vi "Ageing_Loop.vi"(6 "Step Array In":i32[](array[numeric]), 8 "Input Array 2":string[](array[string]), 9 "Input Array 1":string[](array[string])) -> (0 "Step Array Out":i32[](array[numeric]), 1 "True/False":i16, 2 "Output Array 2":string[](array[string]), 3 "Output Array 1":string[](array[string]))   [LabVIEW 2014]
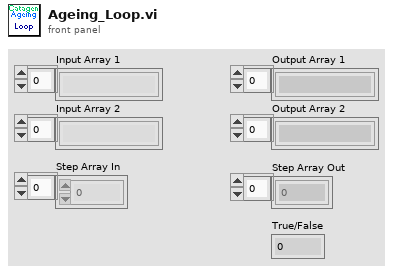
[diagram p1: front panel]
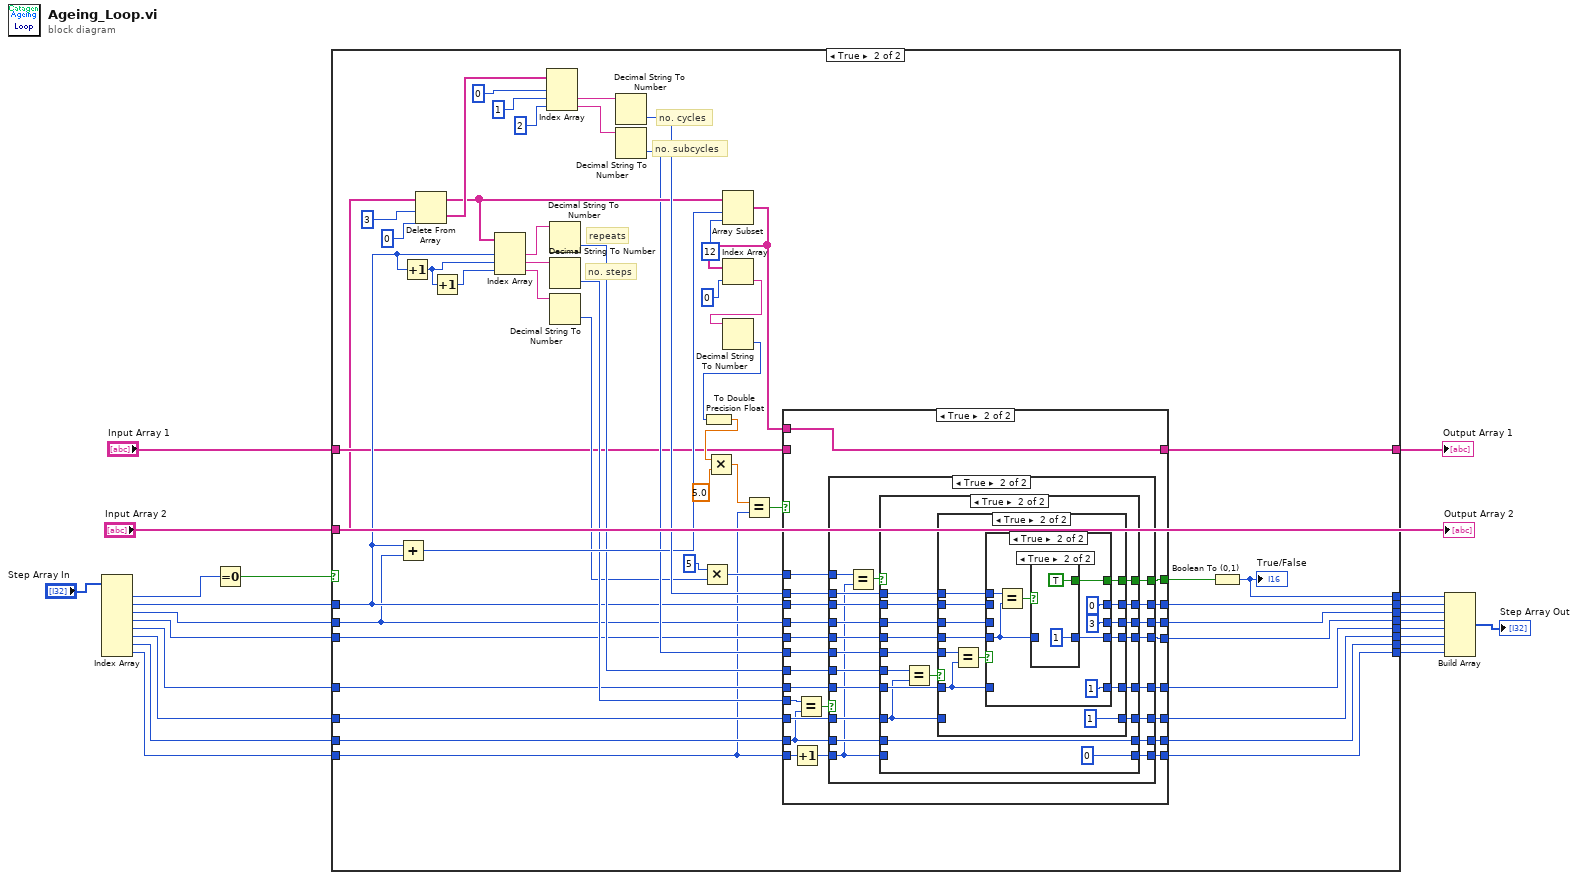
[diagram p0: block diagram]
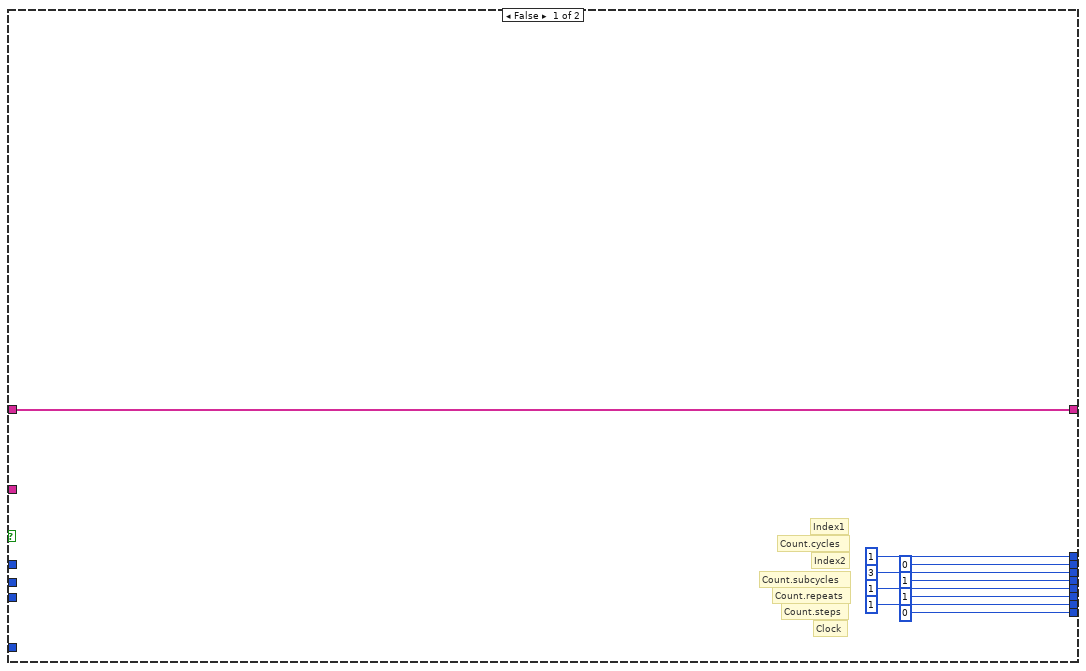
[diagram p2: hidden frame]
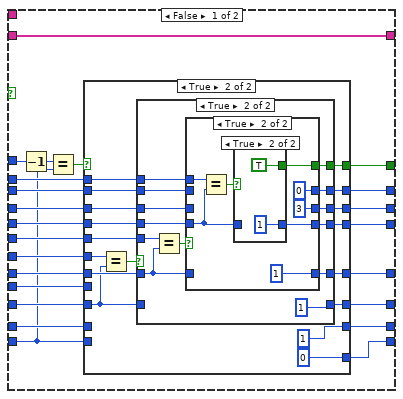
[diagram p3: hidden frame]
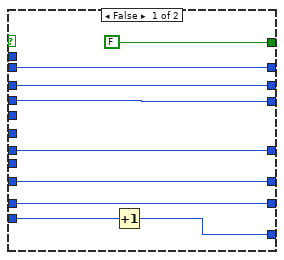
[diagram p4: hidden frame]
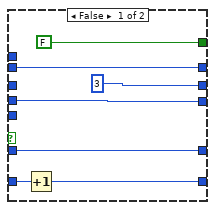
[diagram p5: hidden frame]
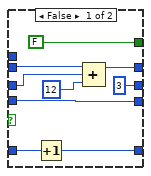
[diagram p6: hidden frame]
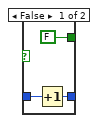
[diagram p7: hidden frame]
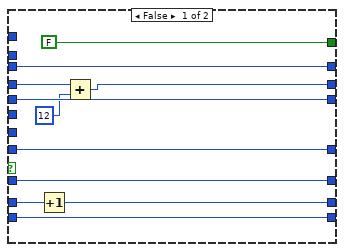
[diagram p8: hidden frame]
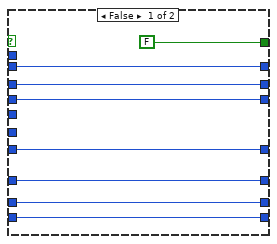
[diagram p9: hidden frame]
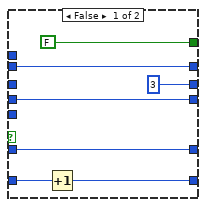
[diagram p10: hidden frame]
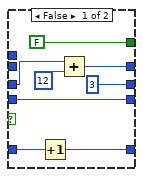
[diagram p11: hidden frame]
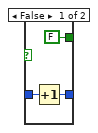
[diagram p12: hidden frame]
diagram:
  n1 = Index Array(array="Step Array In") -> (element #1=w2:i32, element #2=w14:i32, element #3=w13:i32, element #4=w12:i32, element #5=w11:i32, element #6=w10:i32, element #7=w9:i32, element #8=w8:i32)  [unwired: 8 in]
  n2 = Equal To 0?(x=w2) -> (x = 0?=w1:bool)
  n3 = case shown="True" w1 {
    tunnel: [w23 w57] -> w22
    tunnel: [0 w48] -> w21
    tunnel: [3 w47] -> w20
    tunnel: [1 w46] -> w19
    tunnel: [1 w45] -> w18
    tunnel: [1 w44] -> w17
    tunnel: [1 w43] -> w16
    tunnel: [0 w42] -> w15
    tunnel: w14 -> [_ w41]
    tunnel: w13 -> [_ w40]
    tunnel: w12 -> [_ w39]
    tunnel: w11 -> [_ w38]
    tunnel: w10 -> [_ w37]
    tunnel: w9 -> [_ w36]
    tunnel: w8 -> [_ w35]
    tunnel: "Input Array 1" -> [w23 w34]
    tunnel: "Input Array 2" -> [_ w33]
    tunnel: [i16 1 w32] -> w3
    frame False {
      # "Index2"
      # "Index1"
      # "Clock"
      # "Count.steps"
      # "Count.repeats"
      # "Count.subcycles"
      # "Count.cycles"
    }
    frame True {
      # "repeats"
      # "no. steps"
      # "no. subcycles"
      # "no. cycles"
      n4 = Add(x=w41, y=w40) -> (x+y=w67:i32)
      n5 = Increment(x=w41) -> (x+1=w59:i32)
      n6 = Delete From Array(array=w33, length=3, index=0) -> (deleted portion=w76:string[], array with subset deleted=w69:string[])
      n7 = Increment(x=w59) -> (x+1=w58:i32)
      n8 = Index Array(array=w69, index #1=w41, index #2=w59, index #3=w58) -> (element #1=w71:string, element #2=w72:string, element #3=w73:string)
      n9 = Index Array(array=w76, index #1=0 ("index"), index #2=1 ("index"), index #3=2 ("index")) -> (element #2=w75:string, element #3=w74:string)  [unwired: 1 out]
      n10 = Decimal String To Number(string=w71) -> (number=w60:i32)  [unwired: 2 in, 1 out]
      n11 = Decimal String To Number(string=w72) -> (number=w61:i32)  [unwired: 2 in, 1 out]
      n12 = Decimal String To Number(string=w73) -> (number=w49:i32)  [unwired: 2 in, 1 out]
      n13 = Decimal String To Number(string=w75) -> (number=w70:i32)  [unwired: 2 in, 1 out]
      n14 = Decimal String To Number(string=w74) -> (number=w62:i32)  [unwired: 2 in, 1 out]
      n15 = Multiply(x=5, y=w49) -> (x*y=w55:i32)
      n16 = Array Subset(array=w69, index=w67, length=12) -> (w65:string[])
      n17 = Index Array(array=w65, index=0) -> (element=w66:string)
      n18 = Decimal String To Number(string=w66) -> (number=w56:i32)  [unwired: 2 in, 1 out]
      n19 = To Double Precision Float(number=w56) -> (double precision float=w53:dbl)
      n20 = Multiply(x=w53, y=5.0) -> (x*y=w52:dbl)
      n21 = Equal?(x=w52, y=w35) -> (x = y?=w63:bool)
      n22 = case shown="True" w63 {
        tunnel: w40 -> [w94 w195]
        tunnel: [w101 w194] -> w47
        tunnel: w35 -> [w85 w175]
        tunnel: [w96 w180] -> w42
        tunnel: w38 -> [w90 w189]
        tunnel: w36 -> [w88 w176]
        tunnel: [w87 w179] -> w43
        tunnel: w61 -> [w86 w192]
        tunnel: w41 -> [w89 w181]
        tunnel: w37 -> [w97 w177]
        tunnel: [w98 w183] -> w44
        tunnel: w60 -> [w91 w190]
        tunnel: [w99 w184] -> w45
        tunnel: w62 -> [w92 w188]
        tunnel: w39 -> [w93 w187]
        tunnel: w70 -> [w95 w186]
        tunnel: [w100 w185] -> w46
        tunnel: [w102 w182] -> w48
        tunnel: [w104 w193] -> w50
        tunnel: w55 -> [w82 w178]
        tunnel: [w84 w173] -> w57
        tunnel: w34 -> [w84 _]
        tunnel: w65 -> [_ w173]
        frame False {
          n23 = Decrement(x=w82) -> (x-1=w83:i32)
          n24 = Equal?(x=w83, y=w85) -> (x = y?=w103:bool)
          n25 = case shown="True" w103 {
            tunnel: w97 -> [w106 w117]
            tunnel: w91 -> [_ w130]
            tunnel: w90 -> [w105 w128]
            tunnel: w92 -> [_ w127]
            tunnel: w93 -> [w110 w126]
            tunnel: w95 -> [_ w125]
            tunnel: [FALSE w124] -> w104
            tunnel: [w110 w120] -> w100
            tunnel: [w105 w118] -> w99
            tunnel: [w106 w116] -> w98
            tunnel: [w112 w123] -> w102
            tunnel: w94 -> [w111 w122]
            tunnel: [w111 w121] -> w101
            tunnel: w89 -> [w112 w119]
            tunnel: [w108 0] -> w96
            tunnel: w85 -> [w109 _]
            tunnel: w88 -> [w107 _]
            tunnel: [w107 1] -> w87
            tunnel: w86 -> [_ _]
            frame False {
              n26 = Increment(x=w109) -> (x+1=w108:i32)
            }
            frame True {
              n27 = Equal?(x=w130, y=w117) -> (x = y?=w129:bool)
              n28 = case shown="True" w129 {
                tunnel: w128 -> [w132 w140]
                tunnel: w127 -> [_ w150]
                tunnel: w126 -> [w133 w148]
                tunnel: w125 -> [_ w147]
                tunnel: [FALSE w146] -> w124
                tunnel: [w136 w145] -> w123
                tunnel: w122 -> [_ w144]
                tunnel: [3 w143] -> w121
                tunnel: [w133 w142] -> w120
                tunnel: w119 -> [w136 w141]
                tunnel: [w132 w139] -> w118
                tunnel: w117 -> [w135 _]
                tunnel: [w134 1] -> w116
                frame False {
                  n29 = Increment(x=w135) -> (x+1=w134:i32)
                }
                frame True {
                  n30 = Equal?(x=w150, y=w140) -> (x = y?=w149:bool)
                  n31 = case shown="True" w149 {
                    tunnel: w148 -> [w155 w163]
                    tunnel: w147 -> [_ w167]
                    tunnel: [FALSE w165] -> w146
                    tunnel: [w154 0] -> w145
                    tunnel: w144 -> [w152 _]
                    tunnel: [3 ("y") 3] -> w143
                    tunnel: [w155 w164] -> w142
                    tunnel: w141 -> [w151 _]
                    tunnel: w140 -> [w158 _]
                    tunnel: [w157 1] -> w139
                    frame False {
                      n32 = Increment(x=w158) -> (x+1=w157:i32)
                      n33 = Compound Arithmetic op=ADD(w151, w152, 12 ("y")) -> (w154:i32)
                    }
                    frame True {
                      n34 = Equal?(x=w167, y=w163) -> (x = y?=w166:bool)
                      n35 = case shown="True" w166 {
                        tunnel: [FALSE TRUE] -> w165
                        tunnel: [w168 1] -> w164
                        tunnel: w163 -> [w169 _]
                        frame False {
                          n36 = Increment(x=w169) -> (x+1=w168:i32)
                        }
                        frame True {
                        }
                      }
                    }
                  }
                }
              }
            }
          }
        }
        frame True {
          n37 = Increment(x=w175) -> (x+1=w174:i32)
          n38 = Equal?(x=w192, y=w176) -> (x = y?=w191:bool)
          n39 = case shown="True" w191 {
            tunnel: w195 -> [w197 w213]
            tunnel: [w196 w212] -> w194
            tunnel: [FALSE w218] -> w193
            tunnel: w178 -> [_ w226]
            tunnel: w177 -> [w199 w224]
            tunnel: w190 -> [_ w223]
            tunnel: w189 -> [w202 w222]
            tunnel: w188 -> [_ w221]
            tunnel: w187 -> [w203 w220]
            tunnel: w186 -> [_ w219]
            tunnel: w174 -> [w205 w207]
            tunnel: [w203 w217] -> w185
            tunnel: [w202 w216] -> w184
            tunnel: [w199 w215] -> w183
            tunnel: [w204 w214] -> w182
            tunnel: w181 -> [w204 w211]
            tunnel: [w205 w210] -> w180
            tunnel: w176 -> [w201 w208]
            tunnel: [w200 w209] -> w179
            frame False {
              n40 = Increment(x=w201) -> (x+1=w200:i32)
              n41 = Add(x=w197, y=12) -> (x+y=w196:i32)
            }
            frame True {
              n42 = Equal?(x=w226, y=w207) -> (x = y?=w225:bool)
              n43 = case shown="True" w225 {
                tunnel: w224 -> [w232 w238]
                tunnel: w223 -> [_ w251]
                tunnel: w222 -> [w233 w249]
                tunnel: w221 -> [_ w248]
                tunnel: w220 -> [w234 w247]
                tunnel: w219 -> [_ w246]
                tunnel: [FALSE w245] -> w218
                tunnel: [w234 w241] -> w217
                tunnel: [w233 w239] -> w216
                tunnel: [w232 w237] -> w215
                tunnel: [w229 w244] -> w214
                tunnel: w213 -> [w228 w243]
                tunnel: [w228 w242] -> w212
                tunnel: w211 -> [w229 w240]
                tunnel: [w230 0] -> w210
                tunnel: w207 -> [w230 _]
                tunnel: [w227 w235] -> w209
                tunnel: w208 -> [w227 w235]
                frame False {
                }
                frame True {
                  n44 = Equal?(x=w251, y=w238) -> (x = y?=w250:bool)
                  n45 = case shown="True" w250 {
                    tunnel: w249 -> [w253 w261]
                    tunnel: w248 -> [_ w271]
                    tunnel: w247 -> [w254 w269]
                    tunnel: w246 -> [_ w268]
                    tunnel: [FALSE w267] -> w245
                    tunnel: [w257 w266] -> w244
                    tunnel: w243 -> [_ w265]
                    tunnel: [3 ("y") w264] -> w242
                    tunnel: [w254 w263] -> w241
                    tunnel: w240 -> [w257 w262]
                    tunnel: [w253 w260] -> w239
                    tunnel: w238 -> [w256 _]
                    tunnel: [w255 1] -> w237
                    frame False {
                      n46 = Increment(x=w256) -> (x+1=w255:i32)
                    }
                    frame True {
                      n47 = Equal?(x=w271, y=w261) -> (x = y?=w270:bool)
                      n48 = case shown="True" w270 {
                        tunnel: w269 -> [w272 w283]
                        tunnel: w268 -> [_ w287]
                        tunnel: [FALSE w285] -> w267
                        tunnel: [w279 0] -> w266
                        tunnel: w265 -> [w278 _]
                        tunnel: [3 ("y") 3] -> w264
                        tunnel: [w272 w284] -> w263
                        tunnel: w262 -> [_ _]
                        tunnel: w261 -> [w275 _]
                        tunnel: [w274 1] -> w260
                        frame False {
                          n49 = Increment(x=w275) -> (x+1=w274:i32)
                          n50 = Add(x=w278, y=12) -> (x+y=w279:i32)
                        }
                        frame True {
                          n51 = Equal?(x=w287, y=w283) -> (x = y?=w286:bool)
                          n52 = case shown="True" w286 {
                            tunnel: [FALSE TRUE] -> w285
                            tunnel: [w288 1] -> w284
                            tunnel: w283 -> [w289 _]
                            frame False {
                              n53 = Increment(x=w289) -> (x+1=w288:i32)
                            }
                            frame True {
                            }
                          }
                        }
                      }
                    }
                  }
                }
              }
            }
          }
        }
      }
      n54 = Boolean To (0,1)(Boolean=w50) -> (0, 1=w32:i16)
      "True/False" <- w32
    }
  }
  "Output Array 1" <- w22
  n55 = Build Array(w3, w21, w20, w19, w18, w17, w16, w15) -> (→"Step Array Out":i32[])
  "Output Array 2" <- "Input Array 2"
